vi "Flock_RetrieveFIRSTdataException.vi"(8 "Error In":errorcluster, 11 "Process List":T1) -> (0 "Error Out":errorcluster)   [LabVIEW 2013, in "Flock_RetrieveFIRSTdata.lvlib"]
uses:
  Flock_RetrieveFIRSTdata.lvlib
  Shared Code/AMC/VI Source/CentralProcessMessaging/Flock_Shared_CentralProcessMessaging.lvlib
  Shared Code/AMC/VI Source/Error Handling/Flock_ErrorHandling.lvlib
  Shared Code/AMC/VI Source/LocalProcessMessaging/Flock_Shared_LocalProcessMessaging.lvlib
  Shared Code/AMC/VI Source/ProcessList.ctl
  Shared Code/AMC/VI Source/Flock_Shared_Messaging.lvlib
panel:
  out "resulting string":string
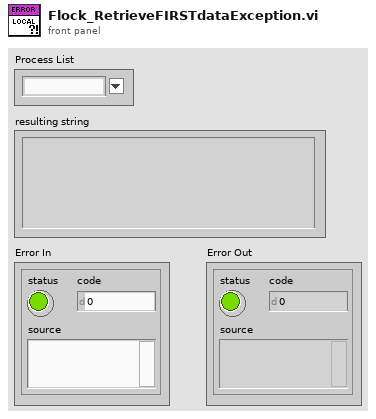
[diagram p1: front panel]
types:
  T1 = typedef "Flock_Shared_Messaging.lvlib/ProcessList.ctl" = string
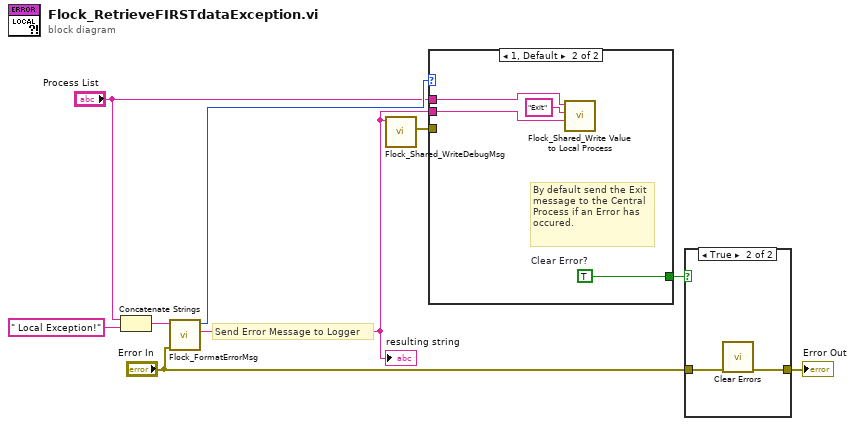
[diagram p0: block diagram]
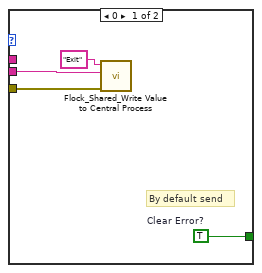
[diagram p3: hidden frame]
diagram:
  # "Send Error Message to Logger"
  n1 = Concatenate Strings("Process List", " Local Exception!" ("initial string")) -> (w1:string)
  n2 = call "Flock_FormatErrorMsg.vi"("error in (no error)"="Error In", "initial string"=w1) -> ("String"=w9:string, "code"=w8:i32)  [unwired: 8 in]
  "resulting string" <- w9
  n3 = call "Flock_Shared_WriteDebugMsg.vi"("Current Message Case"=w9) -> ("error out"=w4:errorcluster)  [unwired: 10 in]
  n4 = case shown="1, Default" w8 {
    tunnel: w9 -> [w12 w15]
    tunnel: [w11 w17] -> w7
    tunnel: w4 -> [w10 _]
    tunnel: "Process List" -> [_ w16]
    frame 0 {
      w11 = TRUE  # Clear Error?
      # "By default send"
      n5 = call "Flock_Shared_Write Value to Central Process.vi"("error in (no error)"=w10, "Message Value"=w12, "Message Name"="Exit") -> ()  [unwired: 8 in, 1 out]
    }
    frame 1, Default {
      w17 = TRUE  # Clear Error?
      # "By default send the Exit message to the Central Process if an Error has occured."
      n6 = call "Flock_Shared_Write Value to Local Process.vi"("Message Value"=w15, "Message Name"="Exit", "Process List"=w16) -> ()  [unwired: 8 in, 1 out]
    }
  }
  n7 = case shown="True" w7 {
    tunnel: "Error In" -> [w18 w20]
    tunnel: [w18 w19] -> w5
    frame False {
    }
    frame True {
      n8 = call <vilib>:"Clear Errors.vi"("error in (no error)"=w20) -> ("error out"=w19:errorcluster)  [unwired: 6 in]
    }
  }
  "Error Out" <- w5
